vi "Fit one.vi"(9 "Initial parameters":dbl[](array[numeric]), 10 "Z":dbl[](array[numeric]), 11 "X":dbl[](array[numeric])) -> ()   [LabVIEW 2016]
uses:
  <vilib>/gmath/NumericalOptimization/Nonlinear Curve Fit LM.vi
  <vilib>/gmath/NI_Gmath.lvlib
panel:
  out "best fit parameters":dbl[](array[numeric])
  out "number of function calls":i32
  in  "termination":cluster{"max iteration":i32, "tolerance":dbl}={"max iteration"=200, "tolerance"=1e-08}
  out "Fit":cluster{"X":dbl[], "best nonlinear fit":dbl[]}[](graph)
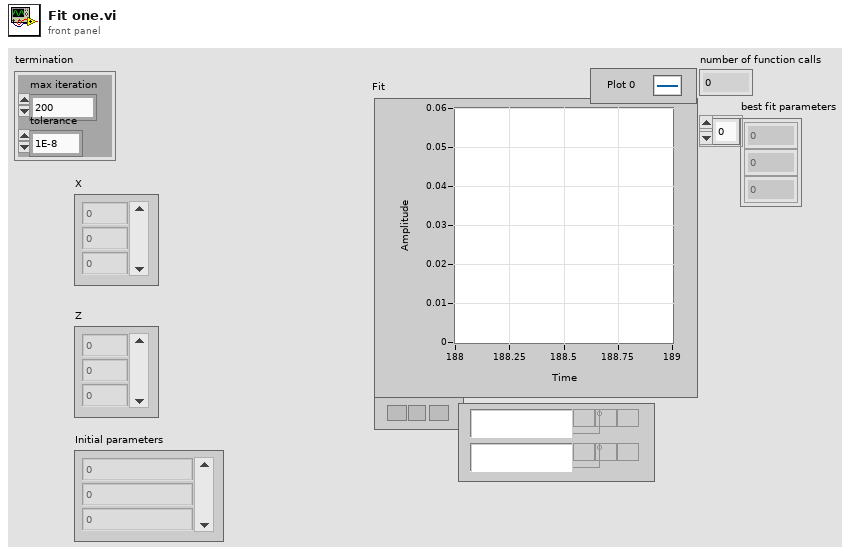
[diagram p1: front panel]
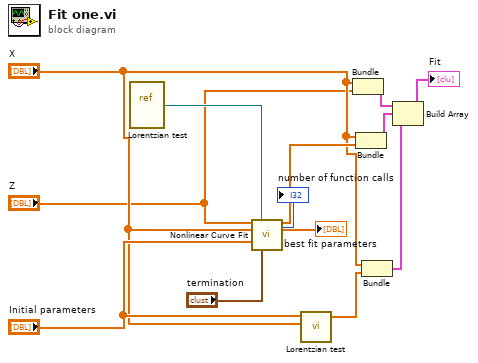
[diagram p0: block diagram]
diagram:
  n1 = vi-ref "Lorentzian test.vi"() -> (w13:refnum<vi>)
  n2 = call-poly <vilib>:"Nonlinear Curve Fit.vi"("Y"="Z", "f(x,a)"=w13, "X"="X", "initial parameters"="Initial parameters", "termination"="termination") -> ("number of function calls"=→"number of function calls":i32, "best nonlinear fit"=w10:dbl[], "best fit parameters"=→"best fit parameters":dbl[])  [unwired: 5 in, 3 out]
  n3 = call "Lorentzian test.vi"("X"="X", "a"="Initial parameters") -> ("f(X,a)"=w3:dbl[])  [unwired: 2 in, 2 out]
  n4 = Bundle("X"="X", "Z"="Z") -> (w12:cluster{"X":dbl[], "Z":dbl[]})  [unwired: 1 in]
  n5 = Bundle("X"="X", "best nonlinear fit"=w10) -> (w11:cluster{"X":dbl[], "best nonlinear fit":dbl[]})  [unwired: 1 in]
  n6 = Bundle("X"="X", "f(X,a)"=w3) -> (w2:cluster{"X":dbl[], "f(X,a)":dbl[]})  [unwired: 1 in]
  n7 = Build Array(w12, w11, w2) -> (→"Fit":cluster{"X":dbl[], "f(X,a)":dbl[]}[])
